vi "Task 2.vi"() -> ()   [LabVIEW 2025]
uses:
  <vilib>/addons/database/Connection.llb/DB Tools Open Connec (String).vi
  <vilib>/addons/database/Connection.llb/Conn Execute.vi
  <vilib>/addons/database/Recordset.llb/Rec Fetch Recordset Data (R).vi
  <vilib>/addons/database/_DB Variant To Data/Database Variant To Data.xnode
  <vilib>/addons/database/NI_Database_API.lvlib
panel:
  in  "search criteria":string
  in  "Multicolumn Listbox":i32(listbox)
  in  "Generate data":bool
  in  "stop":bool
  # "Get data(rows and columns) from SQL server and inserting values to multi column listbox using event strustures"
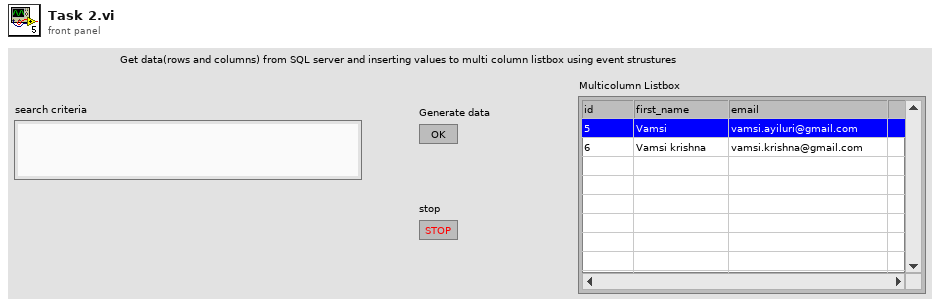
[diagram p1: front panel]
types:
  T1 = typedef "NI_Database_API.lvlib/Conn ObjectReference.ctl" = refnum<k1>
  T2 = typedef "NI_Database_API.lvlib/Rec ObjectReference.ctl" = refnum<k1>
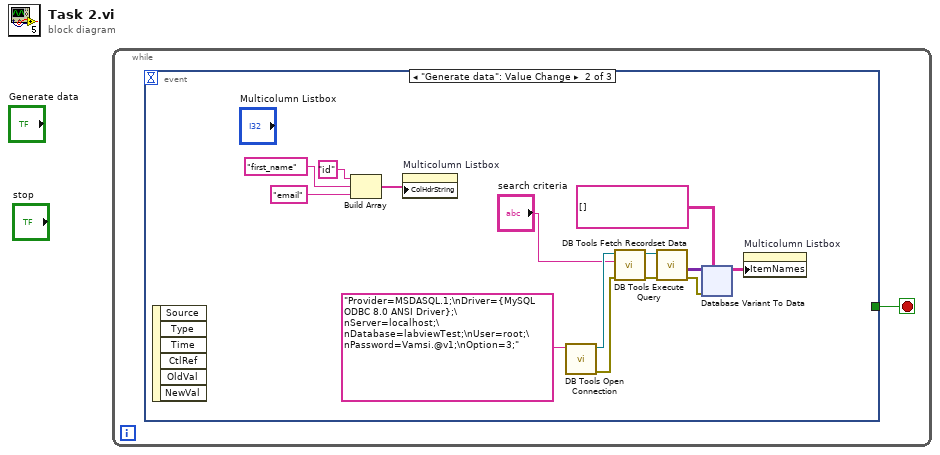
[diagram p0: block diagram]
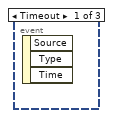
[diagram p2: hidden frame]
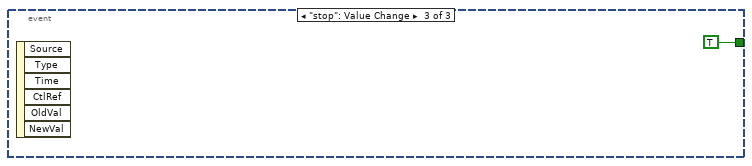
[diagram p3: hidden frame]
diagram:
  n1 = while {
    stop <- w1 stop-if-true
    n2 = event shown="[1] \"Generate data\": Value Change" {
      selector: _ -> [_ _ _]
      dyn-events: _ -> [_ _ _]
      timeout: _ -> [_ _ _]
      tunnel: [_ _ TRUE] -> w1
      event Timeout {
        n3 = event-data() -> ()  [unwired: 1 in, 3 out]
      }
      event "Generate data": Value Change {
        n4 = event-data() -> ()  [unwired: 1 in, 6 out]
        n5 = Build Array("id", "first_name", "email") -> (w10:string[])
        n6 = property on="Multicolumn Listbox" class="MCListbox (strict)"("ColHdrString"=w10) -> ()  [unwired: 2 in, 2 out]
        n7 = call-poly <vilib>:"DB Tools Open Connection.vi"("connection information"="Provider=MSDASQL.1;\nDriver={MySQL ODBC 8.0 ANSI Driver};\nServer=localhost;\nDatabase=labviewTest;\nUser=root;\nPassword=Vamsi.@v1;\nOption=3;") -> ("error out"=w5:errorcluster, "connection reference"=w6:T1)  [unwired: 7 in]
        n8 = call-poly <vilib>:"DB Tools Execute Query.vi"("error in (no error)"=w5, "SQL query"="search criteria", "connection reference"=w6) -> ("error out"=w8:errorcluster, "recordset reference"=w7:T2)  [unwired: 5 in]
        n9 = call-poly <vilib>:"DB Tools Fetch Recordset Data.vi"("error in (no error)"=w8, "recordset reference"=w7) -> ("error out"=w3:errorcluster, "recordset data"=w4:variant[][])  [unwired: 3 in, 1 out]
        n10 = xnode "Database Variant To Data"("database variant"=w4, "error in (no error)"=w3, "type"=string[][] []) -> ("data"=w9:string[][])  [unwired: 1 out]
        n11 = property on="Multicolumn Listbox" class="MCListbox (strict)"("ItemNames"=w9) -> ()  [unwired: 2 in, 2 out]
      }
      event "stop": Value Change {
        n12 = event-data() -> ()  [unwired: 1 in, 6 out]
      }
    }
  }
